vi "Operate.vi"(8 "error in (no error)":errorcluster, 11 "Multiply in":refnum<class "Multiply.lvclass">) -> (0 "error out":errorcluster, 2 "C":dbl, 3 "Multiply out":refnum<class "Multiply.lvclass">)   [LabVIEW 2023, in "Multiply.lvclass"]
uses:
  Multiply.lvclass
  Multiply.lvclass/Multiply.ctl
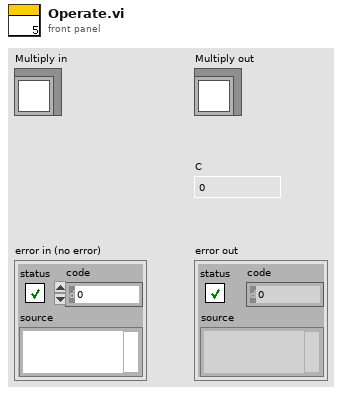
[diagram p1: front panel]
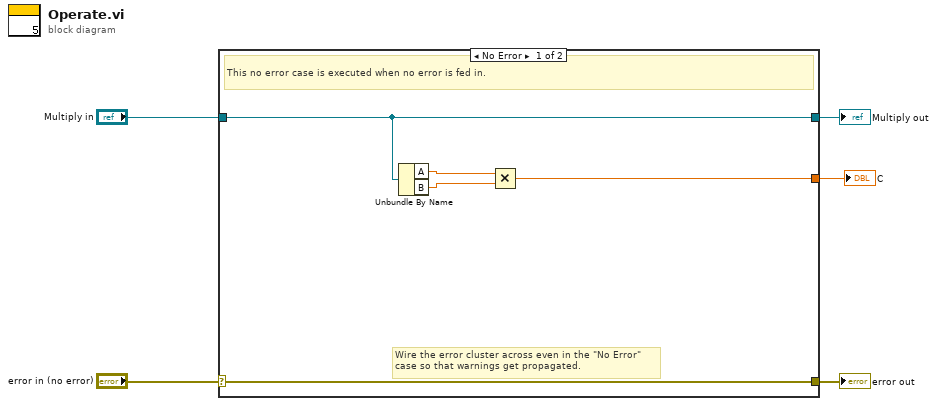
[diagram p0: block diagram]
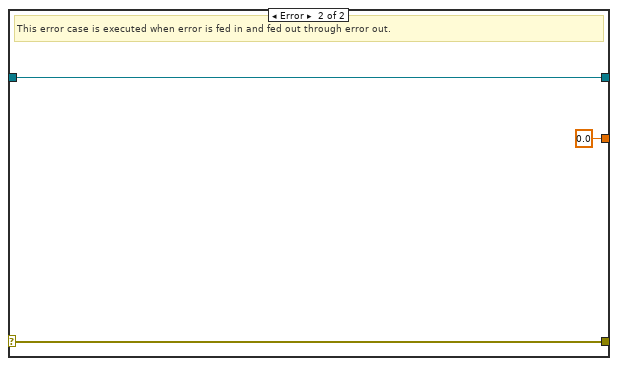
[diagram p2: hidden frame]
diagram:
  n1 = case shown="No Error" "error in (no error)" {
    selector: "error in (no error)" -> [w10 w13]
    tunnel: [w10 w13] -> w4
    tunnel: [w9 w12] -> w2
    tunnel: "Multiply in" -> [w9 w12]
    tunnel: [w6 0.0] -> w1
    frame No Error {
      # "Wire the error cluster across even in the \"No Error\"\ncase so that warnings get propagated."
      # "This no error case is executed when no error is fed in."
      n2 = Unbundle By Name(w9) -> ("A"=w8:dbl, "B"=w7:dbl)
      n3 = Multiply(x=w8, y=w7) -> (x*y=w6:dbl)
    }
    frame Error {
      # "This error case is executed when error is fed in and fed out through error out."
    }
  }
  "error out" <- w4
  "Multiply out" <- w2
  "C" <- w1
